vi "Assign Value.vi"(8 "error in (no error)":errorcluster, 10 "Assigned Value":refnum<class "Abs_Value.lvclass">, 11 "Abs_Boolean_1D in":refnum<class "Abs_Boolean_1D.lvclass">) -> (0 "error out":errorcluster, 3 "Abs_Boolean_1D out":refnum<class "Abs_Boolean_1D.lvclass">)   [LabVIEW 2021, in "Abs_Boolean_1D.lvclass"]
uses:
  Abs_Boolean_1D.lvclass
  Value/Abs_Value.lvclass
  Support/Class Type.ctl
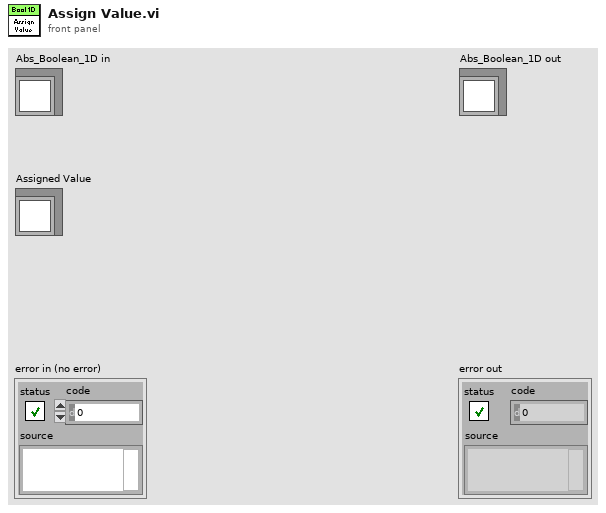
[diagram p1: front panel]
types:
  T1 = typedef "Abs_Boolean_1D.lvclass/Class Type.ctl" = refnum<class "Abs_Boolean_1D.lvclass">
  T2 = typedef "Abs_Boolean_1D.lvclass/Element Type.ctl" = bool
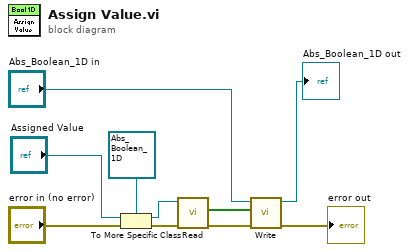
[diagram p0: block diagram]
diagram:
  n1 = To More Specific Class(target class=T1 refnum ("Abs_Boolean_1D.lvclass"), reference="Assigned Value", error in="error in (no error)") -> (specific class reference=w6:T1, error out=w7:errorcluster)
  n2 = call-dynamic "Read.vi"("error in (no error)"=w7, "Boolean in"=w6) -> ("error out"=w5:errorcluster, "Boolean 1D"=w4:T2[])  [unwired: 7 in, 1 out]
  n3 = call-dynamic "Write.vi"("error in (no error)"=w5, "Boolean 1D"=w4, "Boolean in"="Abs_Boolean_1D in") -> ("error out"=→"error out":errorcluster, "Boolean out"=→"Abs_Boolean_1D out":refnum<class "Abs_Boolean_1D.lvclass">)  [unwired: 7 in]
